vi "InitializeAsGRPC.vi"(8 "error in (no error)":errorcluster, 11 "Connection String":string) -> (0 "error out":errorcluster, 2 "MessageUserEvent":refnum<user-event>, 3 "MicronServer":refnum<class "ServiceBase.lvclass">)   [LabVIEW 2019, in "MicronGRPCServer.lvlib" / "GRPCService.lvclass"]
uses:
  GRPCService.lvclass
  Base/Server/Message/MessageBase.lvclass
  Base/Server/Service/ServiceBase.lvclass
  D:/GitHub/KarthikAbiram/Micron/Source/Base/Server/Service/ServiceBase.lvclass
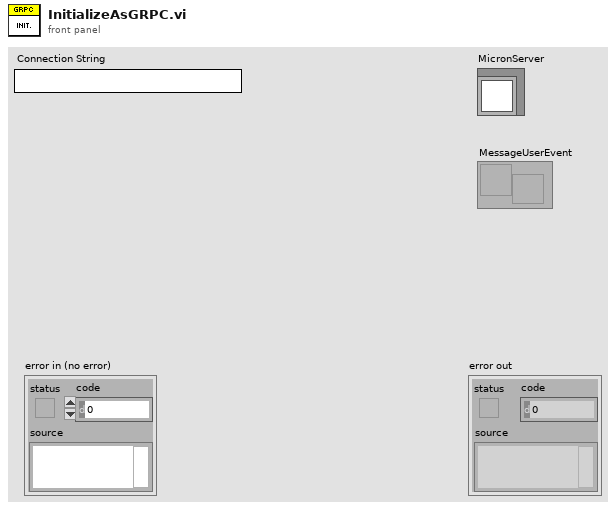
[diagram p1: front panel]
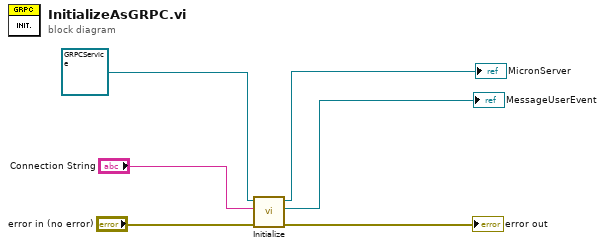
[diagram p0: block diagram]
diagram:
  n1 = call-dynamic "Initialize.vi"("error in (no error)"="error in (no error)", "Connection String"="Connection String", "MicronServer in"=refnum<class "GRPCService.lvclass"> refnum) -> ("error out"=→"error out":errorcluster, "MessageUserEvent"=→"MessageUserEvent":refnum<user-event>, "MicronServer out"=→"MicronServer":refnum<class "GRPCService.lvclass">)  [unwired: 6 in]
